vi "2.A.1-Spoof Centripital Acceleration.vi"(2 "Old Velocity":dbl[](array[numeric]), 3 "Rudder Angle":dbl) -> (0 "Speed":dbl, 1 "New Velocity":dbl[](array[numeric]))   [LabVIEW 2011]
doc: "This vi follows the formula A=([V_old,0]x[0,0,tan(Ra)/.3*norm(V_old)]);\nVnew=norm(V_old)/norm(V_old+A)*(V_old+A)\nThe magic number .3 indicated .3 meters between the rudder and the center of rotation"
uses:
  <vilib>/Analysis/_algsub.llb/Real Vector Norm.vi
  <vilib>/Analysis/NI_AALPro.lvlib
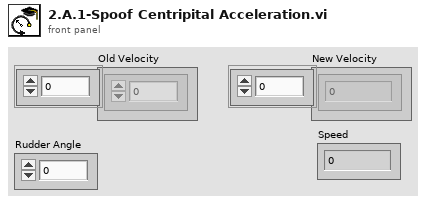
[diagram p1: front panel]
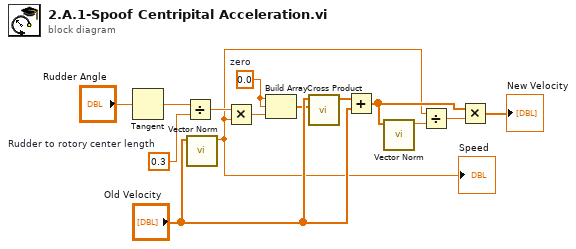
[diagram p0: block diagram]
diagram:
  w10 = 0.0  # zero
  w8 = 0.3  # Rudder to rotory center length
  n1 = Tangent(1:"Rudder Angle") -> (0:w7:dbl)
  n2 = Divide(x=w7, y=w8) -> (x/y=w9:dbl)
  n3 = call-poly <vilib>:"Vector Norm.vi"("Input Vector"="Old Velocity") -> ("norm"=w1:dbl)  [unwired: 9 in, 1 out]
  "Speed" <- w1
  n4 = Multiply(x=w9, y=w1) -> (x*y=w11:dbl)
  n5 = Build Array(w10, w10, w11) -> (w12:dbl[])
  n6 = call <vilib>:"Cross Product.vi"("B Vector"=w12, "A Vector"="Old Velocity") -> ("Cross Product"=w13:dbl[])  [unwired: 8 in, 1 out]
  n7 = Add(x=w13, y="Old Velocity") -> (x+y=w5:dbl[])
  n8 = call-poly <vilib>:"Vector Norm.vi"("Input Vector"=w5) -> ("norm"=w3:dbl)  [unwired: 9 in, 1 out]
  n9 = Divide(x=w1, y=w3) -> (x/y=w2:dbl)
  n10 = Multiply(x=w5, y=w2) -> (x*y=→"New Velocity":dbl[])
